vi "ReadLog.vi"(8 "error in (no error)":errorcluster, 11 "EventRecorder in":refnum<class "EventRecorder.lvclass">) -> (0 "error out":errorcluster, 3 "EventRecorder out":refnum<class "EventRecorder.lvclass">)   [LabVIEW 2019, in "EventRecorder.lvlib" / "EventRecorder.lvclass"]
uses:
  EventRecorder.lvclass
  EventRecorder.lvclass/EventRecorder.ctl
  <vilib>/NI/Event Logger Library/EventLog/Read_CSV.vi
  <vilib>/NI/Event Logger Library/EventLog/EventLog.lvclass
panel:
  out "Description":string
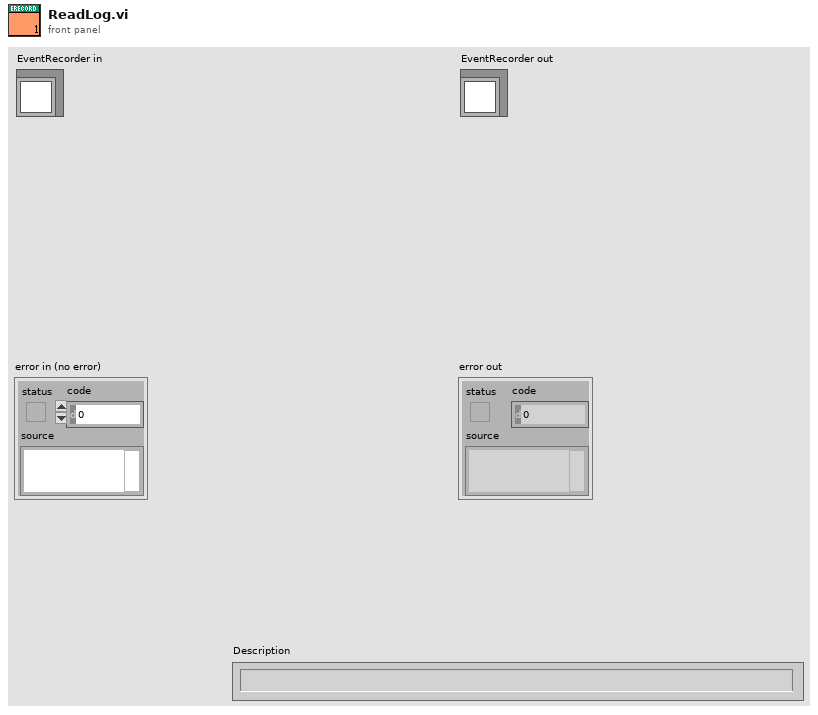
[diagram p1: front panel]
types:
  T1 = typedef "EventBuffer.lvclass/Event_1_0.ctl" = cluster{"TimeStamp":timestamp, "Name":string, "Description":string}
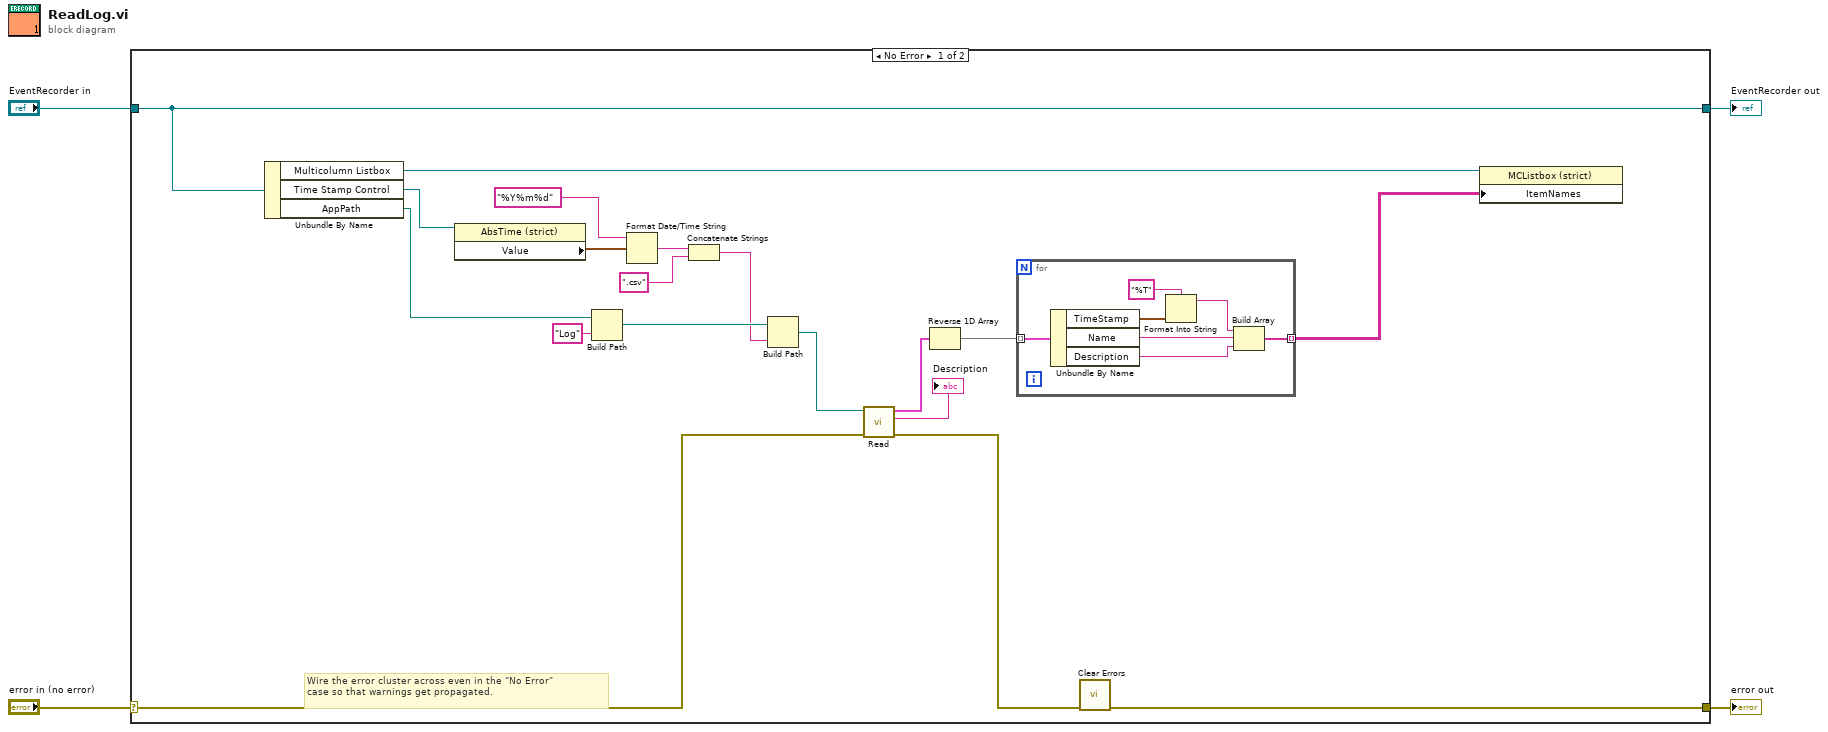
[diagram p0: block diagram]
diagram:
  n1 = case shown="No Error" "error in (no error)" {
    selector: "error in (no error)" -> [w12 w32]
    tunnel: [w5 w32] -> w3
    tunnel: [w20 w31] -> w1
    tunnel: "EventRecorder in" -> [w20 w31]
    frame No Error {
      # "Wire the error cluster across even in the \"No Error\"\ncase so that warnings get propagated."
      n2 = Unbundle By Name(w20) -> ("Multicolumn Listbox"=w19:refnum<vi>, "Time Stamp Control"=w17:refnum<vi>, "AppPath"=w10:path)
      n3 = property class="AbsTime (strict)"(reference=w17) -> ("Value"=w15:timestamp)  [unwired: 1 in, 2 out]
      n4 = Build Path(base path=w10, name or relative path="Log") -> (appended path=w8:path)
      n5 = Format Date/Time String(time format string (%c)="%Y%m%d", seconds (now)=w15) -> (date/time string=w14:string)  [unwired: 1 in]
      n6 = Concatenate Strings(w14, ".csv" ("string")) -> (w7:string)
      n7 = Build Path(base path=w8, name or relative path=w7) -> (appended path=w6:path)
      n8 = call-poly <vilib>:"Read.vi"("error in (no error)"=w12, "Path"=w6) -> ("error out"=w11:errorcluster, "Description"=→"Description":string, "Events"=w22:T1[])  [unwired: 6 in, 1 out]
      n9 = Reverse 1D Array(array=w22) -> (reversed array=w23:T1[])
      n10 = for {
        tunnel: w23 -> [w30] mode=indexing
        tunnel: [w24] -> w18 mode=indexing
        n11 = Unbundle By Name(w30) -> ("TimeStamp"=w29:timestamp, "Name"=w26:string, "Description"=w25:string)
        n12 = Format Into String(format string="%T", w29) -> (resulting string=w27:string)  [unwired: 2 in, 1 out]
        n13 = Build Array(w27, w26, w25) -> (w24:string[])
      }
      n14 = call <vilib>:"Clear Errors.vi"("error in (no error)"=w11) -> ("error out"=w5:errorcluster)  [unwired: 5 in, 1 out]
      n15 = property class="MCListbox (strict)"(reference=w19, "ItemNames"=w18) -> ()  [unwired: 1 in, 2 out]
    }
    frame Error {
    }
  }
  "error out" <- w3
  "EventRecorder out" <- w1
